vi "Open Application Style Reference.vi"(8 "error in (no error)":errorcluster, 11 "ApplicationStyle":refnum<class "IApplicationStyle.lvclass">) -> (0 "error out":errorcluster, 3 "Application Style Reference":T1)   [LabVIEW 2017, in "IViewable.lvlib" / "ApplicationStyleReference.lvclass"]
uses:
  <vilib>/gpm_packages/@cs/mva-viewable/Source/IViewable/ApplicationStyleReference/ApplicationStyleReference.lvclass
  <vilib>/gpm_packages/@cs/mva-viewable/Source/IViewable/IApplicationStyle/IApplicationStyle.lvclass
  <vilib>/gpm_packages/@cs/mva-viewable/Source/IViewable/ApplicationStyleReference/Application Style Reference.ctl
  <vilib>/gpm_packages/@cs/mva-viewable/Source/IViewable/ApplicationStyleReference/ApplicationStyleReference.lvclass/ApplicationStyleReference.ctl
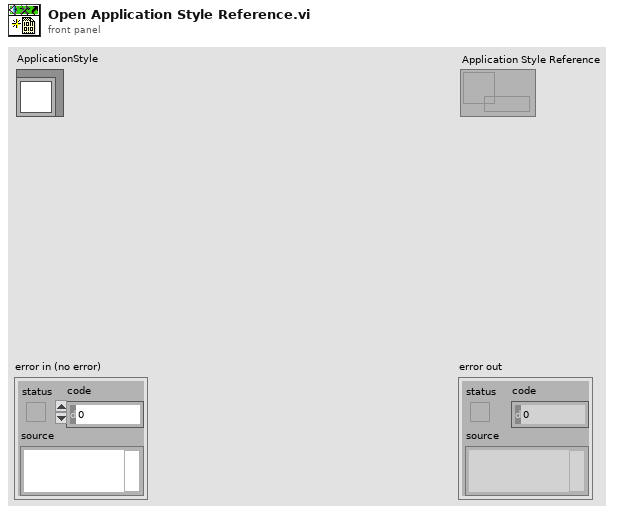
[diagram p1: front panel]
types:
  T1 = typedef "IViewable.lvlib/ApplicationStyleReference.lvclass/Application Style Reference.ctl" = refnum<data-value>
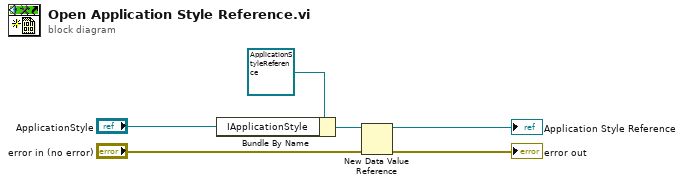
[diagram p0: block diagram]
diagram:
  n1 = Bundle By Name(cluster=refnum<class "ApplicationStyleReference.lvclass"> refnum ("IViewable.lvlib:ApplicationStyleReference.lvclass"), "IApplicationStyle"="ApplicationStyle") -> (w1:refnum<class "ApplicationStyleReference.lvclass">)
  n2 = New Data Value Reference(data value=w1, error in="error in (no error)") -> (data value reference=→"Application Style Reference":refnum<data-value>, error out=→"error out":errorcluster)
